vi "Adb Run Command.vi"(8 "error in (no error)":errorcluster, 10 "args":string, 11 "AdbBridge in":refnum<class "AdbBridge.lvclass">) -> (0 "error out":errorcluster, 3 "AdbBridge out":refnum<class "AdbBridge.lvclass">)   [LabVIEW 2016, in "AdbBridge.lvclass"]
uses:
  AdbBridge.lvclass
  AdbBridge.lvclass/AdbBridge.ctl
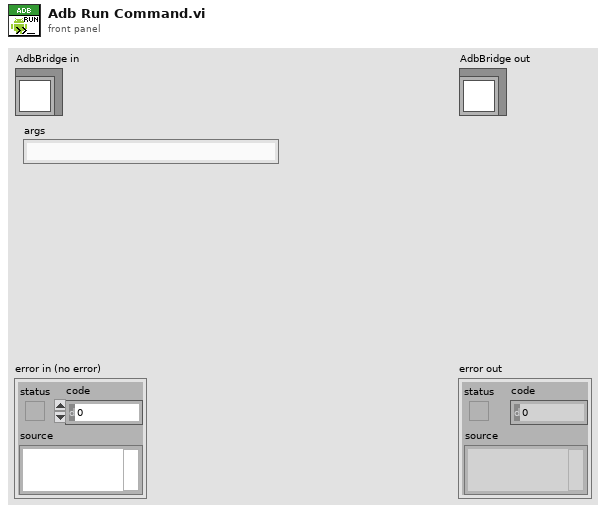
[diagram p1: front panel]
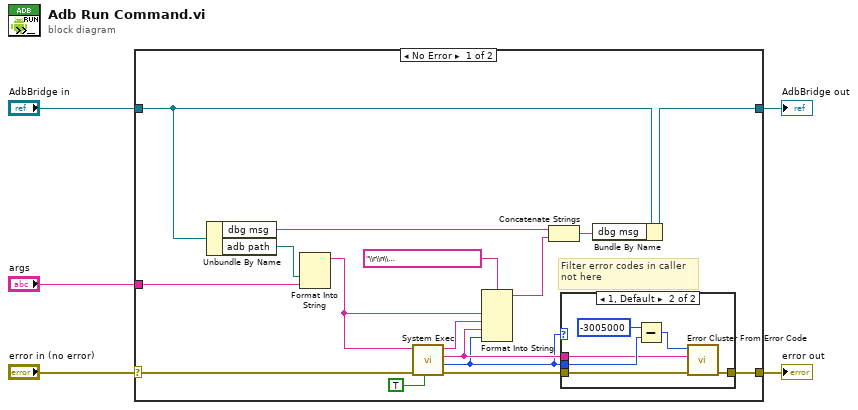
[diagram p0: block diagram]
diagram:
  n1 = case shown="No Error" "error in (no error)" {
    selector: "error in (no error)" -> [w21 w30]
    tunnel: [w8 w30] -> w4
    tunnel: [w15 w29] -> w2
    tunnel: "AdbBridge in" -> [w18 w29]
    tunnel: "args" -> [w16 _]
    frame No Error {
      # "Filter error codes in caller\nnot here"
      n2 = Unbundle By Name(w18) -> ("dbg msg"=w12:string, "adb path"=w17:path)
      n3 = Format Into String(w17, w16) -> (resulting string=w10:string)  [unwired: 3 in, 1 out]
      n4 = call <vilib>:"System Exec.vi"("run minimized? (F)"=TRUE, "error in (no error)"=w21, "command line"=w10) -> ("error out"=w20:errorcluster, "return code"=w6:i32, "standard error"=w7:string, "standard output"=w14:string)  [unwired: 5 in]
      n5 = Format Into String(format string="\\r\\n\\======================\\r\\nRun command: %s \\r\\n stdout: %s \\r\\n stderr: %s \\r\\n errcode: %d", w10, w14, w7, w6) -> (resulting string=w13:string)  [unwired: 2 in, 1 out]
      n6 = Concatenate Strings(w12, w13) -> (w11:string)
      n7 = case shown="1, Default" w6 {
        tunnel: w20 -> [w22 w28]
        tunnel: [w22 w27] -> w8
        tunnel: w6 -> [_ w26]
        tunnel: w7 -> [_ w24]
        frame 0 {
        }
        frame 1, Default {
          n8 = Subtract(x=-3005000, y=w26) -> (x-y=w25:i32)
          n9 = call <vilib>:"Error Cluster From Error Code.vi"("error in (no error)"=w28, "error message (\"\")"=w24, "error code (0)"=w25) -> ("error out"=w27:errorcluster)  [unwired: 6 in]
        }
      }
      n10 = Bundle By Name(cluster=w18, "dbg msg"=w11) -> (w15:refnum<class "AdbBridge.lvclass">)
    }
    frame Error {
    }
  }
  "error out" <- w4
  "AdbBridge out" <- w2
